vi "t1.1.vi"() -> ()   [LabVIEW 2021]
panel:
  out "X":dbl
  out "Y":dbl
  out "Numeric":i32
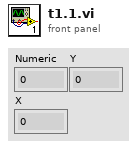
[diagram p1: front panel]
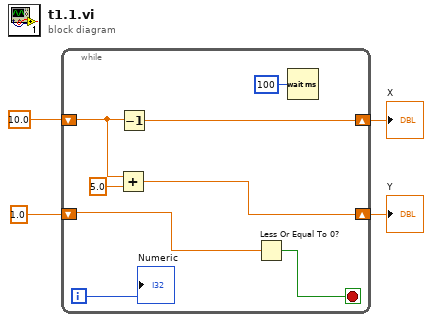
[diagram p0: block diagram]
diagram:
  n1 = while {
    shift-right: [w12] -> w2
    shift-left: 10.0 ("x") -> [w10]
    shift-right: [w9] -> w3
    shift-left: 1.0 -> [w7]
    i -> [w8]
    stop <- w6 stop-if-true
    n2 = Add(x=w10, y=5.0) -> (x+y=w9:dbl)
    n3 = Decrement(x=w10) -> (x-1=w12:dbl)
    n4 = Less Or Equal To 0?(x=w7) -> (x <= 0?=w6:bool)
    n5 = Wait (ms)(milliseconds to wait=u32 100) -> ()  [unwired: 1 out]
    "Numeric" <- w8
  }
  "Y" <- w3
  "X" <- w2
